vi "Periodic Tasks.vi"(8 "error in":errorcluster) -> ()   [LabVIEW 2017]
doc: "This VI runs in parallel to other tasks. It can contain as many user-defined periodic loops as you need. These can carry out PID or other sorts of timed response."
uses:
  Systems/Climber/Climber.lvlib
  Systems/Sonar/Sonar.lvlib
  Systems/VisionSystem/VisionSystem.lvlib
  Systems/Controller/Controller.lvlib
  Systems/MechamumDrive/MechamunDrive.lvlib
  Systems/Hopper/Hopper System.lvlib
  Systems/Intake/Intake.lvlib
  Systems/Shooter/Shooter.lvlib
  Systems/Gear/Gear.lvlib
  Systems/DashBoardCom/DashBoardCom.lvlib
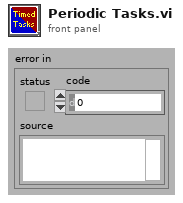
[diagram p1: front panel]
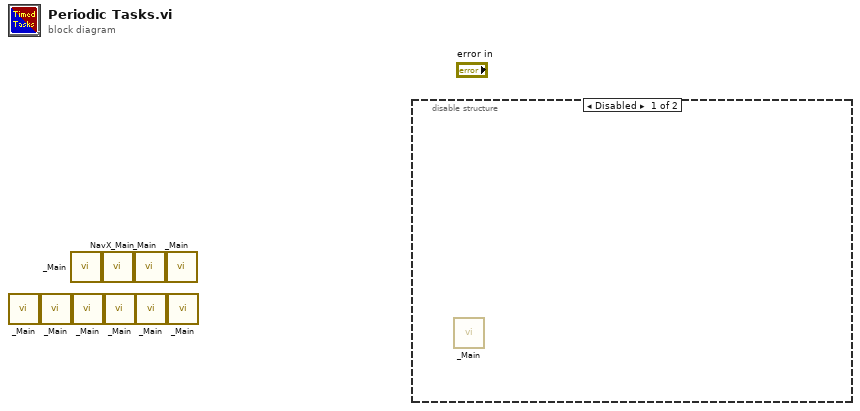
[diagram p0: block diagram]
diagram:
  n1 = call "_Main.vi"() -> ()  [unwired: 12 in]
  n2 = call "_Main.vi"() -> ()  [unwired: 12 in]
  n3 = call "_Main.vi"() -> ()  [unwired: 12 in]
  n4 = call "_Main.vi"() -> ()  [unwired: 12 in]
  n5 = call "NavX_Main.vi"() -> ()  [unwired: 12 in]
  n6 = call "_Main.vi"() -> ()  [unwired: 12 in]
  n7 = call "_Main.vi"() -> ()  [unwired: 12 in]
  n8 = call "_Main.vi"() -> ()  [unwired: 12 in]
  n9 = call "_Main.vi"() -> ()  [unwired: 12 in]
  n10 = call "_Main.vi"() -> ()  [unwired: 12 in]
  n11 = disable-structure shown="Disabled" {
    frame Disabled {
      n12 = call "_Main.vi"() -> ()  [unwired: 12 in]
    }
    frame Enabled {
    }
  }
